vi "Read Controls.vi"(9 "Pane in":refnum<class "Pane.lvclass">) -> (3 "Pane out":refnum<class "Pane.lvclass">, 4 "Controls":refnum<class "Control.lvclass">[](array[class]))   [LabVIEW 2014, in "Pane.lvclass"]
uses:
  Pane.lvclass
  Control/Control.lvclass
  Pane.lvclass/Pane.ctl
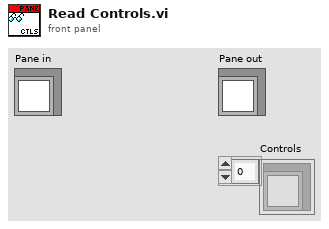
[diagram p1: front panel]
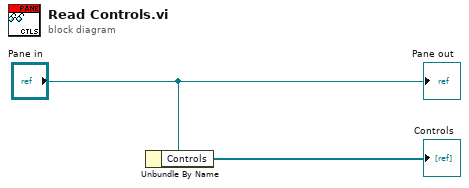
[diagram p0: block diagram]
diagram:
  n1 = Unbundle By Name("Pane in") -> ("Controls"=→"Controls":refnum<class "Control.lvclass">[])
  "Pane out" <- "Pane in"
